vi "Local MS Auto.vi"() -> ()   [LabVIEW 2016]
uses:
  <vilib>/Platform/TimedLoop/XDataNode/timing_clust.ctl
  <vilib>/Platform/TimedLoop/XDataNode/nitl_modes.ctl
  <vilib>/Platform/TimedLoop/XDataNode/wakeup.ctl
  Subsystems/Global Variables.vi
  <vilib>/FPGAPlugInAG/PXI-7833R/niLvFpga_Open_PXI-7833R.vi
  <vilib>/Utility/error.llb/Error Cluster From Error Code.vi
  <vilib>/rvi/errors/niLvFpgaAdjustHostInterfaceError.vi
  <vilib>/FPGAPlugInAG/PXI-7833R/niLvFpga_Reset_PXI-7833R.vi
  <vilib>/FPGAPlugInAG/PXI-7833R/niLvFpga_Close_PXI-7833R.vi
  <vilib>/rvi/interface/nirviOpenFPGA/nirviOpenFPGA.xnode
  FPGA Bitfiles/PhantomControlPI_FPGATarget_QuadCtr2_E2412E44.lvbitx
  IRISS_FPGA_IO.vi
  <vilib>/rvi/interface/nirviReadWriteControl/nirviReadWriteControl.xnode
  <vilib>/platform/TimedLoop/XDataNode/XDataNode.xnode
  <vilib>/rvi/interface/nirviMethod/nirviMethod.xnode
  <vilib>/rvi/interface/nirviCloseFPGA/nirviCloseFPGA.xnode
  Library/KevinLibraryAll/labview2011/kevLib2011.lvlib
  NiFpgaLv.dll
  <vilib>/Platform/TimedLoop/XDataNode/XDNodeRunTimeDep.lvlib
panel:
  out "Pressure Reading":dbl[](array[numeric]) caption="IOP Output [mmHg]"
  in  "Pause":bool caption="To M/S"
  out "Trajectory Cluster":T1
  out "Update Mdl & Traj":bool=TRUE
  out "Stage PID Cluster":T2={"Stage Z PID"={"Kp"=0.0005, "Kd"=0.001, "Ki"=0.0}, "Stage Y PID"={"Kp"=0.0003, "Kd"=0.01, "Ki"=0.0}, "Stage X PID"={"Kp"=0.0003, "Kd"=0.01, "Ki"=0.0}}
  out "L1 to L4 PID Cluster":T3={"L1 PID Gains"={"Kp"=0.005, "Kd"=0.5, "Ki"=0.0005}, "L2 PID Gains"={"Kp"=0.01, "Kd"=1.0, "Ki"=0.0005}, "L3 PID Gains"={"Kp"=0.05, "Kd"=1.0, "Ki"=0.0005}, "L4 PID Gains"={"Kp"=0.1, "Kd"=1.0, "Ki"=0.0005}}
  in  "IRISS GUI":T4(tab)
  in  "OCT Direction":bool
  out "OCT Z out [mm]":dbl caption="OCT Out Z [mm]" format="%#.4f"
  out "X Stage out [mm] 2":dbl caption="Stage X [mm]" format="%#.4f"
  out "Z Stage out [mm] 2":dbl caption="Stage Z [mm]" format="%#.4f"
  out "Y Stage out [mm] 2":dbl caption="Stage Y [mm]" format="%#.4f"
  out "Vacuum Force [mmHg]  2":i32 caption="[mmHg]"
  out "Finished Late Counts":u16
  in  "L2 PID Gains":cluster{"Kp":dbl, "Kd":dbl, "Ki":dbl}={"Kp"=0.01, "Kd"=1.0, "Ki"=0.005}
  in  "L3 PID Gains":cluster{"Kp":dbl, "Kd":dbl, "Ki":dbl}={"Kp"=0.05, "Kd"=1.0, "Ki"=0.0005}
  in  "L4 PID Gains":cluster{"Kp":dbl, "Kd":dbl, "Ki":dbl}={"Kp"=0.1, "Kd"=0.1, "Ki"=0.0005}
  in  "L1 PID Gains":cluster{"Kp":dbl, "Kd":dbl, "Ki":dbl}={"Kp"=0.01, "Kd"=0.5, "Ki"=0.001}
  out "Current System State":T5(ring)
  out "State changing":bool
  out "Tip out Posit":dbl[](array[numeric]) caption="Position [mm]" format="%#.3f"
  out "Tip cmd Posit":dbl[](array[numeric]) caption="Command [mm]" format="%#.3f"
  out "L4 out Posit":dbl caption="y [deg]" format="%#.2g"
  out "L4 cmd Posit":dbl caption="r [deg]" format="%#.2g"
  out "L3 out Posit":dbl caption="y [mm]" format="%#.2g"
  out "L3 cmd Posit":dbl caption="r [mm]" format="%#.2g"
  out "L2 out Posit":dbl caption="y [deg]" format="%#.2g"
  out "L2 cmd Posit":dbl caption="r [deg]" format="%#.2g"
  out "L1 out Posit":dbl caption="y [deg]" format="%#.2g"
  out "L1 cmd Posit":dbl caption="r [deg]" format="%#.2g"
  out "State Flag Array":bool[](array[boolean])
  out "Irrigation Engaged? 2":bool caption="Irrigation Engaged"
  out "OCT Z cmd [mm]":dbl=6.0 caption="OCT Z Ref [mm]" min=0.0 max=12.0 step=0.5
  in  "OCT Z PID Gains":cluster{"Kp":dbl, "Kd":dbl, "Ki":dbl}={"Kp"=0.0003, "Kd"=0.0001, "Ki"=0.01}
  in  "L1 [deg]":dbl
  in  "L2 [deg]":dbl
  in  "L3 [mm]":dbl step=0.1
  in  "L4 [deg]":dbl
  in  "OCT Cmd  [mm]":dbl
  out "Current No.":u8
  in  "No. Cycles":u8=1
  in  "Joint Limits":dbl[][](array[numeric])=[[-8.0, 50.0], [-35.0, 35.0], [-5.0, 20.0], [-180.0, 180.0]] format="%#.3g"
  out "First Trk Pt":dbl[](array[numeric]) format="%#.3g"
  in  "Offset Home 2 RCM":dbl[](array[numeric])=[-7.7, 37.0, 55.0, 0.0] format="%#.3g"
  out "Error(s) Out on Program End":errorcluster
  out "L4 Chart":dbl(graph)
  out "L3 Chart":dbl(graph)
  out "L2 Chart":dbl(graph)
  out "L1 Chart":dbl(graph)
  out "Vac Input":sgl
  in  "Vacuum Step":bool
  in  "Clear Charts":bool
  out "AC Pressure [mmHg]":sgl
  in  "Take IOP Data":bool
  in  "Irrigation":bool
  in  "PID ON/OFF":bool
  in  "Vac PID Gains":cluster{"Kp":dbl, "Kd":dbl, "Ki":dbl, "Ts":dbl}={"Kp"=5.0, "Kd"=0.0, "Ki"=5.0, "Ts"=0.01}
  in  "Vac Cmd":sgl min=0 max=100 step=1 format="%#_13g"
  in  "Target IOP":sgl=20.0 min=0 max=100 step=1 format="%#_13g"
  out "IOP Ctrl":T6(graph)
  out "Pressure Sensors":T7(graph)
  in  "Reset Joystick":bool caption="Encoder Reset"
  in  "Max Limit [mmHg]":dbl=600.0
  in  "Increase":bool
  in  "Vac Step Size":sgl=50.0 min=0 max=100 step=1 format="%#_13g"
  in  "Wait Time [ms]":i32=200
  out "Vacuum":sgl
  out "Irrigation":sgl
  in  "Hydration":bool
  out "Z Stage out [mm]":dbl caption="Output Z [mm]" format="%#.4f"
  out "Z Stage cmd [mm]":dbl=6.0 caption="Reference Z [mm]" min=0.0 max=12.0 step=0.5
  out "Y Stage out [mm]":dbl caption="Output Y [mm]" format="%#.4f"
  out "Y Stage cmd [mm]":dbl=6.0 caption="Reference Y  [mm]" min=0.0 max=12.0 step=0.5
  out "X Stage out [mm]":dbl caption="Output X [mm]" format="%#.4f"
  out "X Stage cmd [mm]":dbl=6.0 caption="Reference X [mm]" min=0.0 max=12.0 step=0.5
  in  "Stage Z PID Gains":cluster{"Kp":dbl, "Kd":dbl, "Ki":dbl}={"Kp"=0.0005, "Kd"=0.001, "Ki"=0.0}
  in  "Stage Y PID Gains":cluster{"Kp":dbl, "Kd":dbl, "Ki":dbl}={"Kp"=0.0001, "Kd"=0.005, "Ki"=0.0}
  in  "Stage X PID Gains":cluster{"Kp":dbl, "Kd":dbl, "Ki":dbl}={"Kp"=0.0003, "Kd"=0.01, "Ki"=0.0}
  out "Irrigation Engaged?":bool
  out "Accurus Button":bool[](array[boolean]) caption="Remote Button Command"
  out "Voltage Output Ch. B":dbl(graph)
  out "Voltage Output Ch. A":dbl(graph)
  out "Accurus Engaged?":bool
  out "Vacuum Force [mmHg]":i32
  in  "Load Traj":bool caption="To M/S"
  in  "Retract":bool caption="To M/S"
  in  "Stop Accurus":bool caption="To M/S"
  in  "L3 Go Home":bool caption="To M/S"
  in  "Track":bool caption="To M/S"
  in  "Program Stop":bool
  # "Robot Status"
  # "OCT"
  # "Tool Tip Location"
  # "L1"
  # "X\nY\nZ"
  # "X\nY\nZ"
  # "+"
  # "_"
  # "L2"
  # "Reserved"
  # "System Progress"
  # "L3"
  # "Homing finished"
  # "Reserved"
  # "M/S initialization finished"
  # "Trajecoty loading finished"
  # "L4"
  # "Tracking initialization finished"
  # "In Tracking"
  # "Notes: \n2. check state transition\n4. preview trajectory?"
  # "Vacuum"
  # "Joint Motion"
  # "Calibration"
  # "Space Deform Parameters"
  # "L1"
  # "[deg]"
  # "L2"
  # "[deg]"
  # "L3"
  # "[mm]"
  # "L4"
  # "[deg]"
  # "First Track Point"
  # "AC & PC Gap"
  # "L1"
  # "[deg]"
  # "L2"
  # "[deg]"
  # "L3"
  # "[mm]"
  # "L4"
  # "[deg]"
  # "Error Message"
  # "Tracking Joint Limits"
  # "Incision"
  # "Min."
  # "Max."
  # "L1"
  # "L1"
  # "[deg]"
  # "L2"
  # "L2"
  # "[deg]"
  # "L3"
  # "L3"
  # "[mm]"
  # "L4"
  # "L4"
  # "[deg]"
  # "Data Saving"
  # "Vacuum Profile"
  # "IOP Feedback Control"
  # "Eye Hydration"
  # "XYZ Stage Control"
  # "OCT Z-Axis"
  # "Moved to main tab"
  # "Foot Pedal Buttons"
  # "Irrigation and Aspiration"
  # "Button 1"
  # "Button 2"
  # "Button 3"
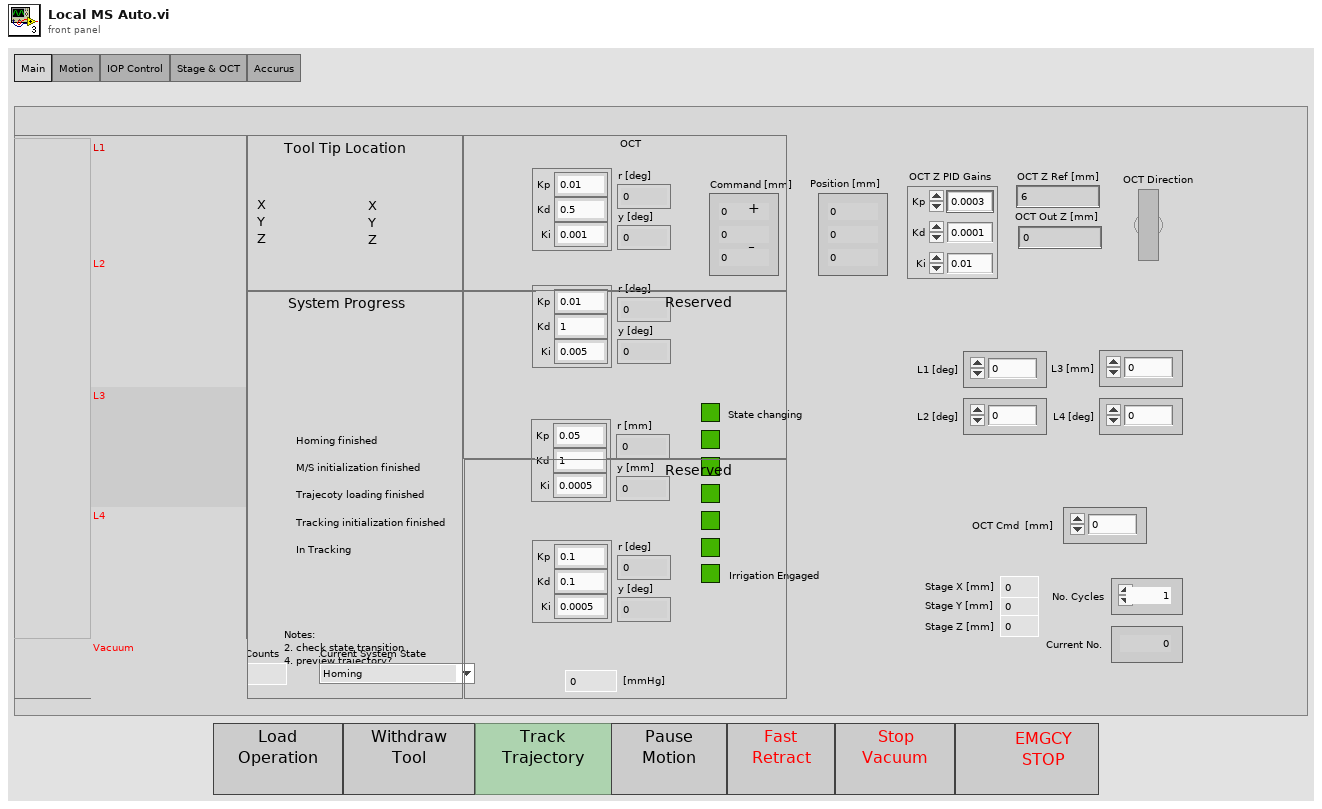
[diagram p1: front panel]
types:
  T1 = cluster{"Traj Px Array":dbl[], "Traj Py Array":dbl[], "Traj Pz Array":dbl[]}
  T2 = cluster{"Stage Z PID":cluster{"Kp":dbl, "Kd":dbl, "Ki":dbl}, "Stage Y PID":cluster{"Kp":dbl, "Kd":dbl, "Ki":dbl}, "Stage X PID":cluster{"Kp":dbl, "Kd":dbl, "Ki":dbl}}
  T3 = cluster{"L1 PID Gains":cluster{"Kp":dbl, "Kd":dbl, "Ki":dbl}, "L2 PID Gains":cluster{"Kp":dbl, "Kd":dbl, "Ki":dbl}, "L3 PID Gains":cluster{"Kp":dbl, "Kd":dbl, "Ki":dbl}, "L4 PID Gains":cluster{"Kp":dbl, "Kd":dbl, "Ki":dbl}}
  T4 = enum32{"Main", "Motion", "IOP Control", "Stage & OCT", "Accurus"}
  T5 = enum16{"Homing", "M/S Initialization", "M/S Operation", "Trajectory Loading", "Tracking Initialization", "Tracking"}
  T6 = cluster{"[0]":dbl, "[1]":dbl, "[2]":dbl, "[3]":dbl, "[4]":dbl, "[5]":dbl, "[6]":dbl, "[7]":dbl, "[8]":dbl}
  T7 = cluster{"Pressure Reading[0]":dbl, "Pressure Reading[1]":dbl, "Pressure Reading[2]":dbl, "Pressure Reading[3]":dbl, "Pressure Reading[4]":dbl, "Pressure Reading[5]":dbl, "Pressure Reading[6]":dbl, "Pressure Reading[7]":dbl, "Pressure Reading[8]":dbl}
  T8 = cluster{"Prev L1 to L4 Posit":dbl[], "Prev Stage Posit":dbl[], "Prev OCT Z Posit":dbl}
  T9 = typedef "XDNodeRunTimeDep.lvlib/timing_clust.ctl" = cluster{"Expected End [f-1]":u64, "Actual End [f-1]":u64, "Finished Late? [f-1]":bool, "Expected End [i-1]":u64, "Actual End [i-1]":u64, "Finished Late? [i-1]":bool, "Expected Start [i]":u64, "Actual Start [i]":u64, "Expected Start [f]":u64, "Actual Start [f]":u64, "Source Name":string, "Structure Name":string, "Period":i64, "Deadline":i64, "Offset":i64, "Start":i64, "Priority":i32, "Timeout":i32, "Mode":T10, "Wakeup Reason":T11, "Error":errorcluster, "Source Type":string, "Secondary Source Type":string, "Global End Time":u64, "Global Start Time":u64, "Frame Duration":u64, "Iteration Duration":u64, "Assigned CPU":i32, "I/O Scan Engine Mode":u32}
  T10 = typedef "XDNodeRunTimeDep.lvlib/nitl_modes.ctl" = enum32{"No Change", "Process missed periods, maintain original phase", "Discard missed periods, maintain original phase", "Process missed periods, ignore original phase", "Discard missed periods, ignore original phase"}
  T11 = typedef "XDNodeRunTimeDep.lvlib/wakeup.ctl" = enum32{"Normal", "Aborted", "Asynchronous wakeup", "Timing source error", "Timed loop error", "Timeout"}
  T12 = cluster{"L1 to L4 PID Cluster":cluster{"L1 PID Gains":cluster{"Kp":dbl, "Kd":dbl, "Ki":dbl}, "L2 PID Gains":cluster{"Kp":dbl, "Kd":dbl, "Ki":dbl}, "L3 PID Gains":cluster{"Kp":dbl, "Kd":dbl, "Ki":dbl}, "L4 PID Gains":cluster{"Kp":dbl, "Kd":dbl, "Ki":dbl}}, "Stage PID Cluster":cluster{"Stage Z PID":cluster{"Kp":dbl, "Kd":dbl, "Ki":dbl}, "Stage Y PID":cluster{"Kp":dbl, "Kd":dbl, "Ki":dbl}, "Stage X PID":cluster{"Kp":dbl, "Kd":dbl, "Ki":dbl}}, "OCT Z PID Gains":cluster{"Kp":dbl, "Kd":dbl, "Ki":dbl}}
  T13 = enum8{"Enabled", "Disabled", "Disabled and Grayed Out"}
  T14 = cluster{"Last L1 to L4 Posit":dbl[], "Last Stage Posit":dbl[], "Last OCT Z Posit":dbl}
  T15 = cluster{"Accurus button":bool[], "Accurus engaged?":bool, "Vacuum Force":i32, "Accurus Ch. A Vout":dbl, "Accurus Ch. B Vout":dbl, "Irrigation engaged?":bool}
  T16 = cluster{"pressure sensors[0]":sgl, "pressure sensors[1]":sgl, "pressure sensors[2]":sgl, "pressure sensors[3]":sgl, "pressure sensors[4]":sgl, "pressure sensors[5]":sgl, "pressure sensors[6]":sgl, "pressure sensors[7]":sgl, "pressure sensors[8]":sgl}[]
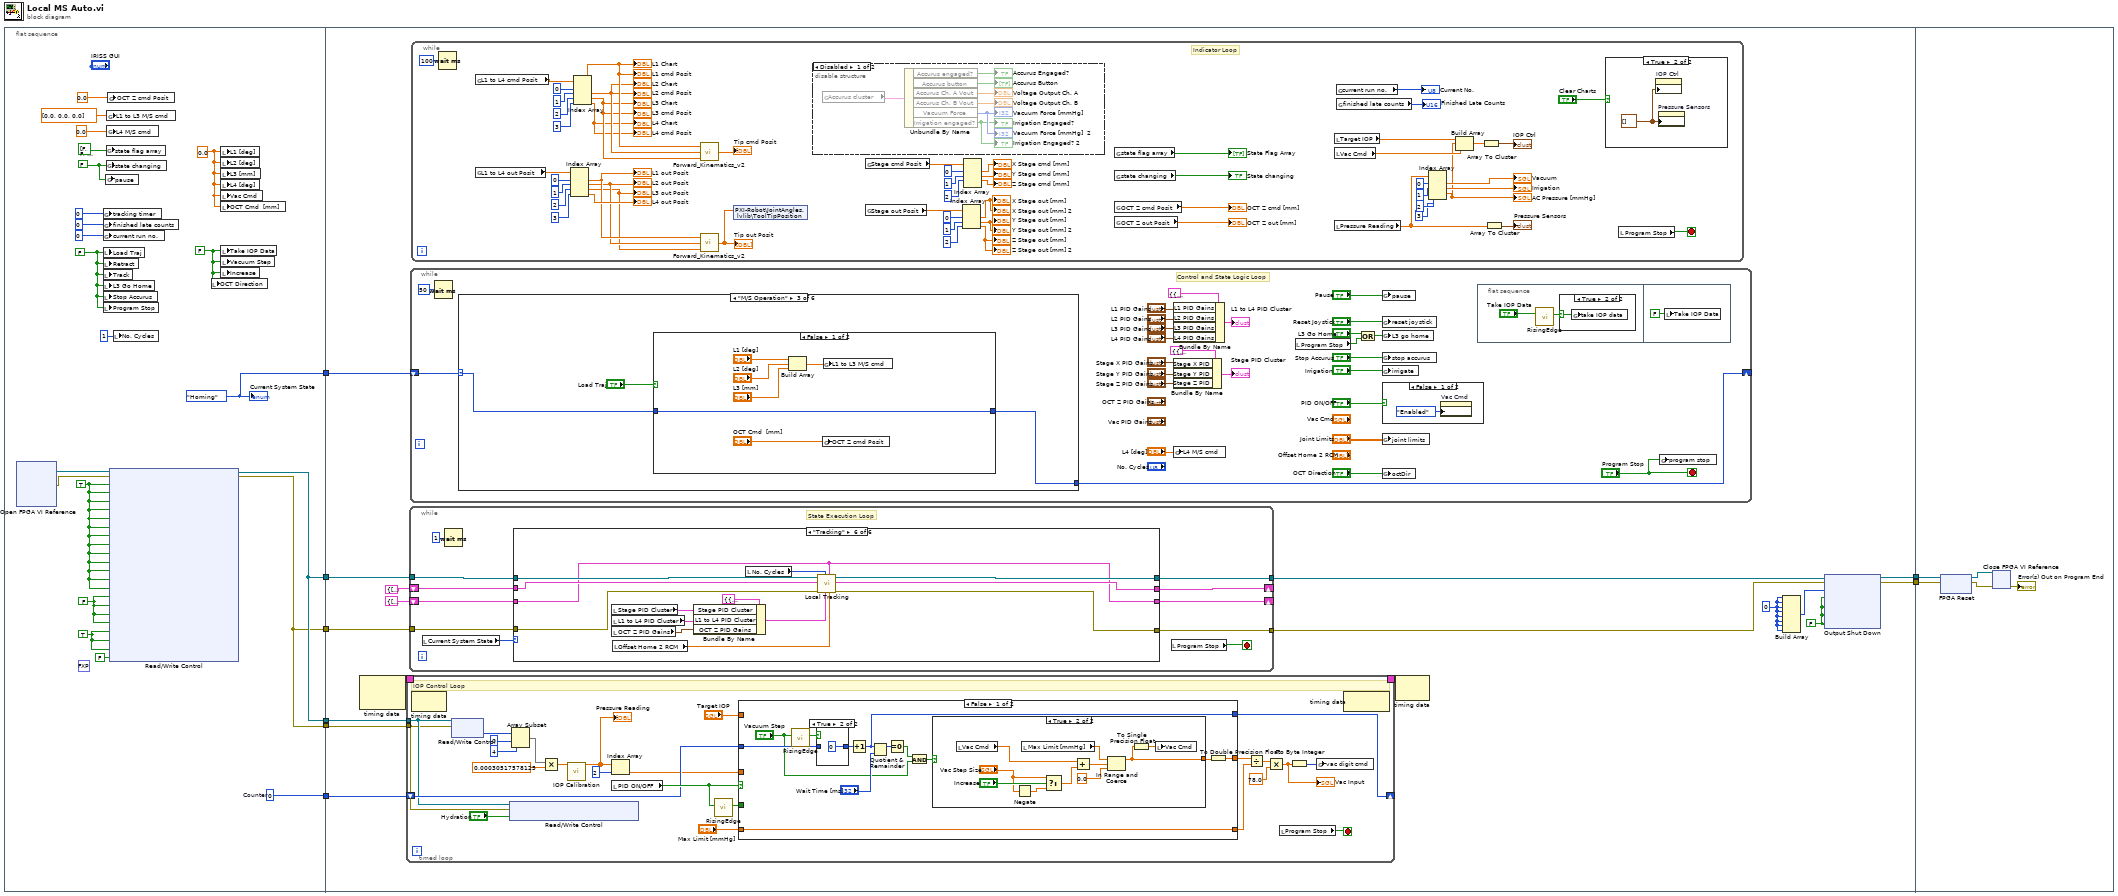
[diagram p0: block diagram]
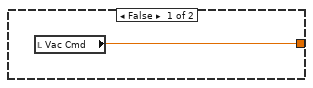
[diagram p3: hidden frame]
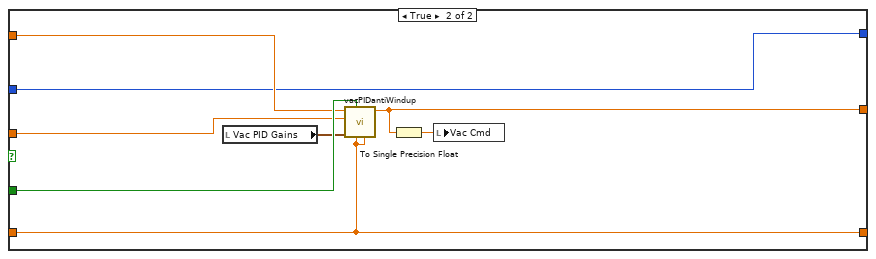
[diagram p4: hidden frame]
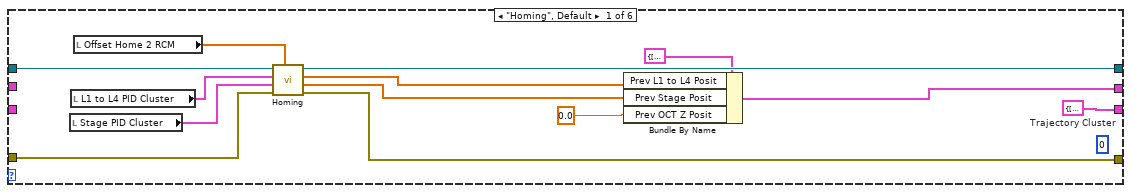
[diagram p7: hidden frame]
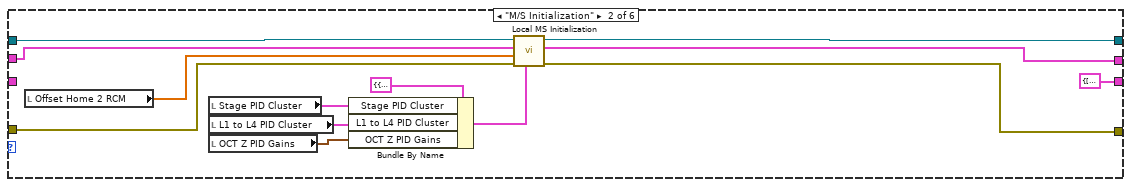
[diagram p8: hidden frame]
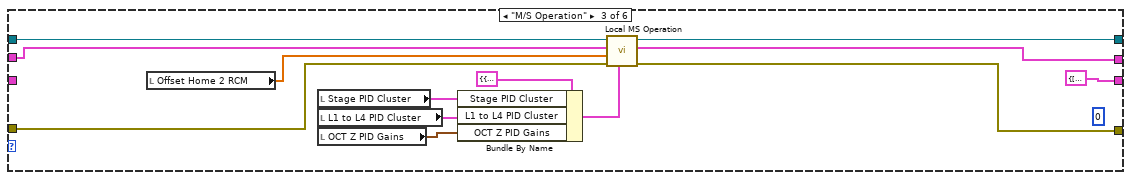
[diagram p9: hidden frame]
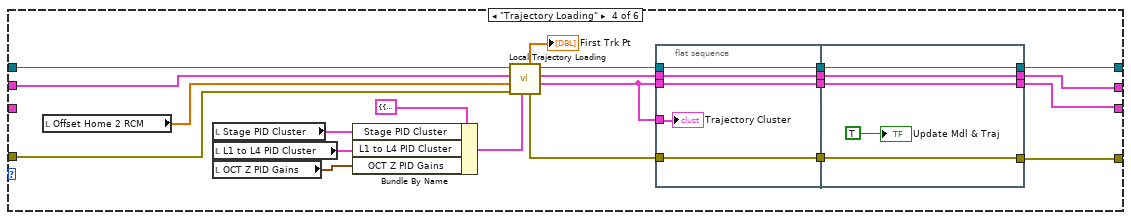
[diagram p10: hidden frame]
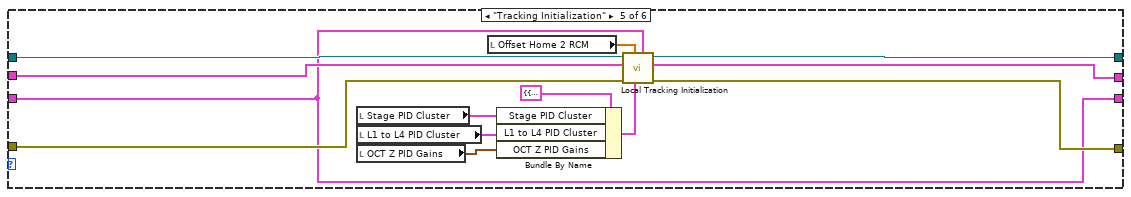
[diagram p11: hidden frame]
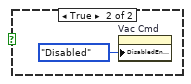
[diagram p13: hidden frame]
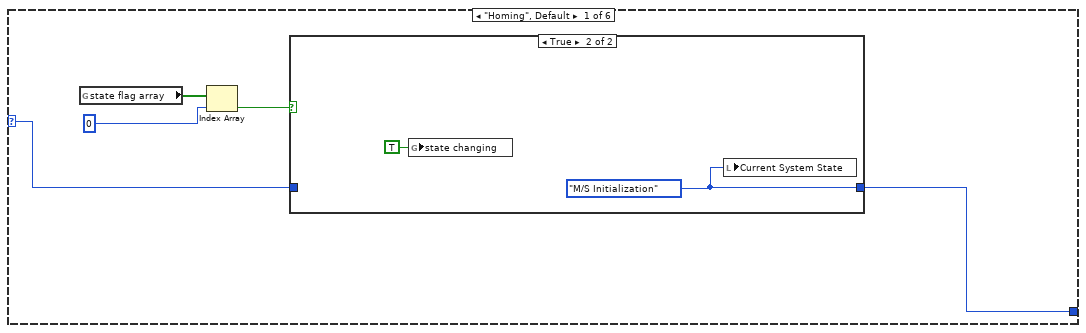
[diagram p14: hidden frame]
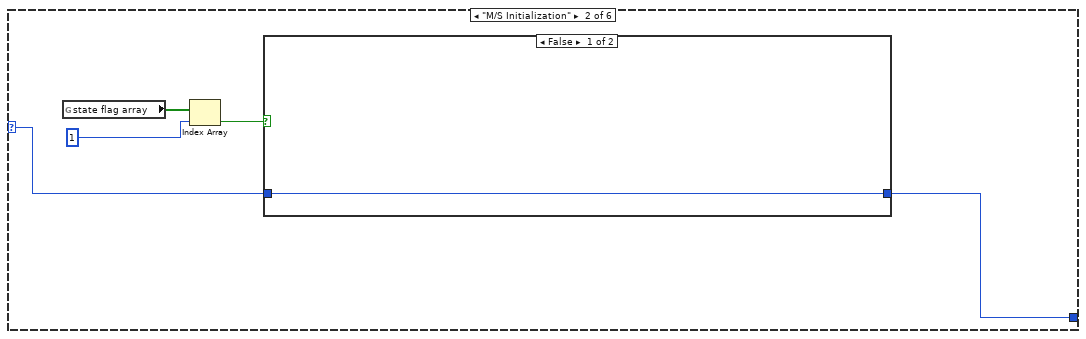
[diagram p16: hidden frame]
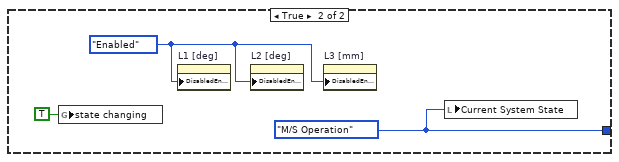
[diagram p17: hidden frame]
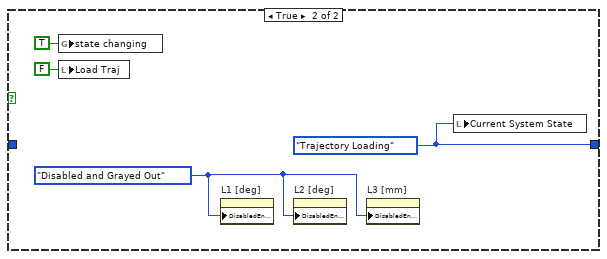
[diagram p18: hidden frame]
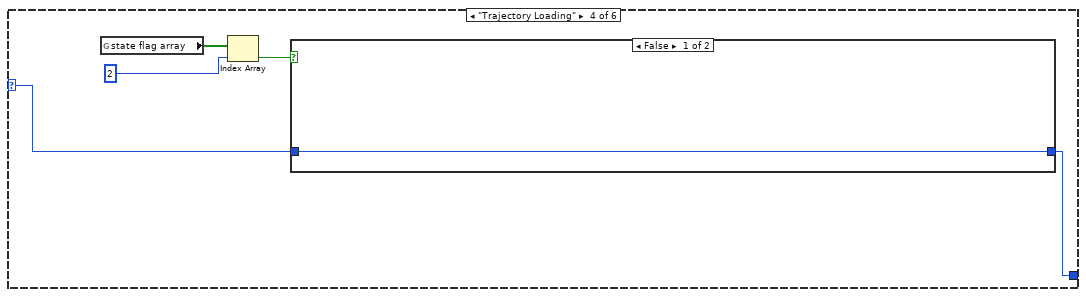
[diagram p19: hidden frame]
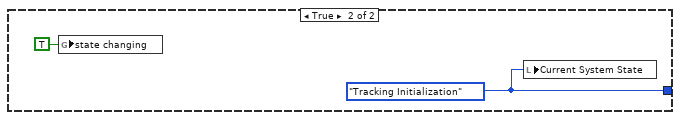
[diagram p20: hidden frame]
diagram:
  n1 = flat-sequence {
    tunnel: [w9] -> w8
    tunnel: [w10] -> w7
    tunnel: [w22] -> w6
    tunnel: [w10] -> w3
    tunnel: [w9] -> w2
    tunnel: [w14] -> w1
    tunnel: w8 -> [w46]
    tunnel: w7 -> [w47]
    tunnel: w6 -> [w38]
    tunnel: [w40] -> w5
    tunnel: [w39] -> w4
    tunnel: w3 -> [w33]
    tunnel: w2 -> [w32]
    tunnel: w1 -> [w31]
    tunnel: w5 -> [w395]
    tunnel: w4 -> [w396]
    frame #0 {
      (unwired) fxp<+,32,0> 0.0 ("Duty Cycle")
      w14 = 0  # Counter
      w11 = FALSE ("Take IOP Data")
      w12 = 0.0 ("L4 M/S cmd")
      w22 = T5."Homing" ("Current State")
      w23 = FALSE ("state changing")
      w29 = TRUE ("Conn0/DIO12 Button 1")
      w28 = FALSE ("Reset")
      w30 = TRUE ("Reset")
      w24 = FALSE ("program stop")
      n2 = xnode "Open FPGA VI Reference"() -> ("FPGA VI Reference Out"=w27:refnum<k20>, "error out"=w26:errorcluster)  [unwired: 2 in]
      n3 = global write "Global Variables.vi" "tracking timer"(0 ("finished late counts")) -> ()
      n4 = global write "Global Variables.vi" "finished late counts"(u16 0 ("finished late counts")) -> ()
      n5 = global write "Global Variables.vi" "current run no."(u8 0 ("current run no.")) -> ()
      n6 = local write "Load Traj"(w24) -> ()
      n7 = local write "Retract"(w24) -> ()
      n8 = local write "Track"(w24) -> ()
      n9 = local write "L3 Go Home"(w24) -> ()
      n10 = local write "Stop Accurus"(w24) -> ()
      n11 = local write "Program Stop"(w24) -> ()
      n12 = global write "Global Variables.vi" "pause"(w23) -> ()
      n13 = global write "Global Variables.vi" "state flag array"(bool[] [FALSE, FALSE, FALSE, FALSE, FALSE, FALSE, FALSE, FALSE, FALSE] ("state flag array")) -> ()
      n14 = global write "Global Variables.vi" "state changing"(w23) -> ()
      n15 = global write "Global Variables.vi" "L1 to L3 M/S cmd"(dbl[] [0.0, 0.0, 0.0] ("L1 to L3 M/S cmd")) -> ()
      n16 = global write "Global Variables.vi" "L4 M/S cmd"(0.0 ("L4 M/S cmd")) -> ()
      n17 = global write "Global Variables.vi" "OCT Z cmd Posit"(0.0 ("L4 M/S cmd")) -> ()
      n18 = xnode "Read/Write Control"("FPGA VI Reference In"=w27, "error in"=w26, "Reset 1"=w30, "Reset 3"=w30, "Reset 9"=w30, "Reset 10"=w30, "Reset 11"=w30, "Reset 12"=w30, "Reset 13"=w30, "Reset 14"=w30, "Reset 15"=w30, "Reset 16"=w30, "Reset 17"=w30, "Reset C1-1"=w30, "Reset C1-4"=w30, "INHB X"=w28, "INHB Y"=w28, "INHB Z"=w28, "INHB OCT Mot"=w28, "Conn0/DIO12 Button 1"=w29, "Conn0/DIO13 Button 2"=w29, "Conn0/DIO15 Button 4"=w29, "Hydration On/Off (Connector2/DIO28)"=FALSE) -> ("FPGA VI Reference Out"=w10:refnum<k20>, "error out"=w9:errorcluster)
      n19 = local write "No. Cycles"(1 ("No. Cycles")) -> ()
      n20 = local write "OCT Direction"(w11) -> ()
      n21 = local write "L1 [deg]"(w12) -> ()
      n22 = local write "L2 [deg]"(w12) -> ()
      n23 = local write "L3 [mm]"(w12) -> ()
      n24 = local write "L4 [deg]"(w12) -> ()
      n25 = local write "Vac Cmd"(w12) -> ()
      n26 = local write "OCT Cmd  [mm]"(w12) -> ()
      n27 = local write "Take IOP Data"(w11) -> ()
      n28 = local write "Vacuum Step"(w11) -> ()
      n29 = local write "Increase"(w11) -> ()
      "Current System State" <- w22
    }
    frame #1 {
      w44 = FALSE
      w37 = i16 0 ("element")
      n30 = node-c288 ("Input Node")() -> (w35:T9)  [unwired: 2 in]
      n31 = timed-loop {
        timing: w35 -> [_]
        timing-out: [_] -> w34
        tunnel: w33 -> [w50]
        tunnel: w32 -> [w49]
        shift-right: [w52] -> _
        shift-left: w31 -> [w53]
        stop <- w63 stop-if-true
        # "IOP Control Loop"
        n32 = node-c288() -> ()  [unwired: 1 in, 1 out]
        n33 = xnode "Read/Write Control"("FPGA VI Reference In"=w50, "error in"=w49) -> ("AI"=w66:i16[])  [unwired: 2 out]
        n34 = xnode "Read/Write Control"("FPGA VI Reference In"=w50, "error in"=w49, "Hydration On/Off (Connector2/DIO28)"="Hydration") -> ()  [unwired: 2 out]
        n35 = Array Subset(array=w66, index=0, length=4) -> (w72:i16[])
        n36 = Multiply(x=w72, y=0.00030517578125) -> (x*y=w56:dbl[])
        n37 = call "IOP Calibration.vi"("IOP Input [V]"=w56) -> ("IOP Output [mmHg]"=w67:dbl[])  [unwired: 10 in]
        "Pressure Reading" <- w67
        n38 = Index Array(array=w67, index=2) -> (element=w48:dbl)
        n39 = local read "PID ON/OFF"() -> (w64:bool)
        n40 = call "RisingEdge.vi"("Signal In"=w64) -> ("Rising Edge"=w65:bool)  [unwired: 10 in]
        n41 = case shown="False" w64 {
          tunnel: w48 -> [_ w101]
          tunnel: "Target IOP" -> [_ w102]
          tunnel: [w84 w105] -> w62
          tunnel: "Max Limit [mmHg]" -> [w83 w104]
          tunnel: [w83 w104] -> w54
          tunnel: w65 -> [_ w103]
          tunnel: w53 -> [w76 w98]
          tunnel: [w73 w98] -> w52
          frame False {
            n42 = call "RisingEdge.vi"("Signal In"="Vacuum Step") -> ("Rising Edge"=w77:bool)  [unwired: 10 in]
            n43 = case shown="True" w77 {
              tunnel: [w85 0] -> w80
              tunnel: w76 -> [w85 _]
              frame False {
              }
              frame True {
              }
            }
            n44 = Increment(x=w80) -> (x+1=w73:i32)
            n45 = Quotient & Remainder(x=w73, y="Wait Time [ms]") -> (x-y*floor(x/y)=w79:i32)  [unwired: 1 out]
            n46 = Equal To 0?(x=w79) -> (x = 0?=w81:bool)
            n47 = And(x=w81, y="Vacuum Step") -> (x .and. y?=w75:bool)
            n48 = case shown="True" w75 {
              tunnel: [w87 w97] -> w82
              frame False {
                n49 = local read "Vac Cmd"() -> (w87:sgl)
              }
              frame True {
                n50 = local read "Vac Cmd"() -> (w90:sgl)
                n51 = Negate(x="Vac Step Size") -> (-x=w88:sgl)
                n52 = local read "Max Limit [mmHg]"() -> (w94:dbl)
                n53 = Select(t="Vac Step Size", s="Increase", f=w88) -> (s? t:f=w92:sgl)
                n54 = Add(x=w90, y=w92) -> (x+y=w96:sgl)
                n55 = In Range and Coerce(upper limit=w94, x=w96, lower limit=0.0 ("y")) -> (coerced(x)=w97:dbl)  [unwired: 1 out]
                n56 = To Single Precision Float(number=w97) -> (single precision float=w91:sgl)
                n57 = local write "Vac Cmd"(w91) -> ()
              }
            }
            n58 = To Double Precision Float(number=w82) -> (double precision float=w84:dbl)
          }
          frame True {
            n59 = local read "Vac PID Gains"() -> (w100:cluster{"Kp":dbl, "Kd":dbl, "Ki":dbl, "Ts":dbl})
            n60 = call "vacPIDantiWindup.vi"("Saturation U"=w104, "Saturation M"=w104, "Reset"=w103, "PID Gains"=w100, "Feedback"=w101, "Reference"=w102) -> ("Control"=w105:dbl)  [unwired: 5 in]
            n61 = To Single Precision Float(number=w105) -> (single precision float=w99:sgl)
            n62 = local write "Vac Cmd"(w99) -> ()
          }
        }
        n63 = Divide(x=w62, y=w54) -> (x/y=w61:dbl)
        n64 = Multiply(x=w61, y=78.0) -> (x*y=w55:dbl)
        "Vac Input" <- w55
        n65 = local read "Program Stop"() -> (w63:bool)
        n66 = To Byte Integer(number=w55) -> (8bit integer=w59:i8)
        n67 = global write "Global Variables.vi" "vac digit cmd"(w59) -> ()
        n68 = node-c288() -> ()  [unwired: 1 in, 1 out]
      }
      n69 = while {
        tunnel: w47 -> [w182]
        tunnel: w46 -> [w181]
        tunnel: [w180] -> w42
        tunnel: [w179] -> w41
        shift-right: [w177] -> _
        shift-left: T8 {"Prev L1 to L4 Posit"=[0.0, 0.0, 0.0, 0.0], "Prev Stage Posit"=[6.0, 6.0, 6.0], "Prev OCT Z Posit"=0.0} ("Prev Posit Cluster") -> [w178]
        shift-right: [w175] -> _
        shift-left: T1 {"Traj Px Array"=[], "Traj Py Array"=[], "Traj Pz Array"=[]} ("Trajectory Cluster") -> [w174]
        stop <- w176 stop-if-true
        # "State Execution Loop"
        n70 = local read "Current System State"() -> (w183:T5)
        n71 = Wait (ms)(milliseconds to wait=u32 1) -> ()  [unwired: 1 out]
        n72 = case shown="\"Tracking\"" w183 {
          tunnel: w182 -> [w197 w210 w223 w245 w268 w282]
          tunnel: w181 -> [w196 w209 w222 w244 w267 w281]
          tunnel: [w195 w208 w221 w227 w266 w280] -> w180
          tunnel: [w194 w207 w220 w233 w265 w279] -> w179
          tunnel: w178 -> [_ w206 w219 w243 w263 w278]
          tunnel: [w193 w205 w218 w232 w264 w277] -> w177
          tunnel: [w185 T1 {"Traj Px Array"=[], "Traj Py Array"=[], "Traj Pz Array"=[]} ("Trajectory Cluster") T1 {"Traj Px Array"=[], "Traj Py Array"=[], "Traj Pz Array"=[]} ("Trajectory Cluster") w225 w256 w271] -> w175
          tunnel: w174 -> [_ _ _ _ w256 w271]
          frame "Homing", Default {
            w185 = T1 {"Traj Px Array"=[], "Traj Py Array"=[], "Traj Pz Array"=[]}  # Trajectory Cluster
            (unwired) 0 ("Last Index")
            n73 = local read "Stage PID Cluster"() -> (w189:T2)
            n74 = local read "L1 to L4 PID Cluster"() -> (w190:T3)
            n75 = local read "Offset Home 2 RCM"() -> (w192:dbl[])
            n76 = call "Homing.vi"("Offset Home 2 RCM"=w192, "error in"=w196, "Stage PID Cluster"=w189, "L1 to L4 PID Cluster"=w190, "FPGA VI Reference In"=w197) -> ("error out"=w194:errorcluster, "Last Stage Posit"=w186:dbl[], "Last L1 to L4 Posit"=w187:dbl[], "FPGA VI Reference Out"=w195:refnum<k20>)  [unwired: 3 in]
            n77 = Bundle By Name(cluster=T8 {"Prev L1 to L4 Posit"=[-0.5409, 0.04404050915429177, -1.917656453185038, 0.02068014705882353], "Prev Stage Posit"=[6.001471972029684, 5.996134588585126, 6.000298217087839], "Prev OCT Z Posit"=-0.0} ("Prev Posit Cluster"), "Prev L1 to L4 Posit"=w187, "Prev Stage Posit"=w186, "Prev OCT Z Posit"=0.0) -> (w193:T8)
          }
          frame "M/S Initialization" {
            n78 = local read "Offset Home 2 RCM"() -> (w199:dbl[])
            n79 = local read "Stage PID Cluster"() -> (w204:T2)
            n80 = local read "L1 to L4 PID Cluster"() -> (w203:T3)
            n81 = local read "OCT Z PID Gains"() -> (w202:cluster{"Kp":dbl, "Kd":dbl, "Ki":dbl})
            n82 = Bundle By Name(cluster=T12 {"L1 to L4 PID Cluster"={"L1 PID Gains"={"Kp"=0.005, "Kd"=0.5, "Ki"=0.0005}, "L2 PID Gains"={"Kp"=0.01, "Kd"=1.0, "Ki"=0.005}, "L3 PID Gains"={"Kp"=0.05, "Kd"=1.0, "Ki"=0.0005}, "L4 PID Gains"={"Kp"=0.1, "Kd"=0.1, "Ki"=0.0005}}, "Stage PID Cluster"={"Stage Z PID"={"Kp"=0.0005, "Kd"=0.001, "Ki"=0.0}, "Stage Y PID"={"Kp"=0.0003, "Kd"=0.01, "Ki"=0.0}, "Stage X PID"={"Kp"=0.0003, "Kd"=0.01, "Ki"=0.0}}, "OCT Z PID Gains"={"Kp"=0.0003, "Kd"=0.0001, "Ki"=0.01}} ("PID Cluster"), "Stage PID Cluster"=w204, "L1 to L4 PID Cluster"=w203, "OCT Z PID Gains"=w202) -> (w200:T12)
            n83 = call "Local MS Initialization.vi"("PID Cluster"=w200, "error in"=w209, "Offset Home 2 RCM"=w199, "Prev Posit Cluster"=w206, "FPGA VI Reference In"=w210) -> ("error out"=w207:errorcluster, "Last Posit Cluster"=w205:T14, "FPGA VI Reference Out"=w208:refnum<k20>)  [unwired: 4 in]
          }
          frame "M/S Operation" {
            (unwired) 0 ("Last Index")
            n84 = local read "Offset Home 2 RCM"() -> (w212:dbl[])
            n85 = local read "Stage PID Cluster"() -> (w217:T2)
            n86 = local read "L1 to L4 PID Cluster"() -> (w216:T3)
            n87 = local read "OCT Z PID Gains"() -> (w215:cluster{"Kp":dbl, "Kd":dbl, "Ki":dbl})
            n88 = Bundle By Name(cluster=T12 {"L1 to L4 PID Cluster"={"L1 PID Gains"={"Kp"=0.005, "Kd"=0.5, "Ki"=0.0005}, "L2 PID Gains"={"Kp"=0.01, "Kd"=1.0, "Ki"=0.005}, "L3 PID Gains"={"Kp"=0.05, "Kd"=1.0, "Ki"=0.0005}, "L4 PID Gains"={"Kp"=0.1, "Kd"=0.1, "Ki"=0.0005}}, "Stage PID Cluster"={"Stage Z PID"={"Kp"=0.0005, "Kd"=0.001, "Ki"=0.0}, "Stage Y PID"={"Kp"=0.0003, "Kd"=0.01, "Ki"=0.0}, "Stage X PID"={"Kp"=0.0003, "Kd"=0.01, "Ki"=0.0}}, "OCT Z PID Gains"={"Kp"=0.0003, "Kd"=0.0001, "Ki"=0.01}} ("PID Cluster"), "Stage PID Cluster"=w217, "L1 to L4 PID Cluster"=w216, "OCT Z PID Gains"=w215) -> (w213:T12)
            n89 = call "Local MS Operation.vi"("PID Cluster"=w213, "error in"=w222, "Offset Home 2 RCM"=w212, "Prev Posit Cluster"=w219, "FPGA VI Reference In"=w223) -> ("error out"=w220:errorcluster, "Last Posit Cluster"=w218:T14, "FPGA VI Reference Out"=w221:refnum<k20>)  [unwired: 4 in]
          }
          frame "Trajectory Loading" {
            n90 = local read "Offset Home 2 RCM"() -> (w237:dbl[])
            n91 = local read "Stage PID Cluster"() -> (w242:T2)
            n92 = local read "L1 to L4 PID Cluster"() -> (w241:T3)
            n93 = local read "OCT Z PID Gains"() -> (w240:cluster{"Kp":dbl, "Kd":dbl, "Ki":dbl})
            n94 = Bundle By Name(cluster=T12 {"L1 to L4 PID Cluster"={"L1 PID Gains"={"Kp"=0.005, "Kd"=0.5, "Ki"=0.0005}, "L2 PID Gains"={"Kp"=0.01, "Kd"=1.0, "Ki"=0.005}, "L3 PID Gains"={"Kp"=0.05, "Kd"=1.0, "Ki"=0.0005}, "L4 PID Gains"={"Kp"=0.1, "Kd"=0.1, "Ki"=0.0005}}, "Stage PID Cluster"={"Stage Z PID"={"Kp"=0.0005, "Kd"=0.001, "Ki"=0.0}, "Stage Y PID"={"Kp"=0.0003, "Kd"=0.01, "Ki"=0.0}, "Stage X PID"={"Kp"=0.0003, "Kd"=0.01, "Ki"=0.0}}, "OCT Z PID Gains"={"Kp"=0.0003, "Kd"=0.0001, "Ki"=0.01}} ("PID Cluster"), "Stage PID Cluster"=w242, "L1 to L4 PID Cluster"=w241, "OCT Z PID Gains"=w240) -> (w238:T12)
            n95 = call "Local Trajectory Loading.vi"("PID Cluster"=w238, "error in"=w244, "Offset Home 2 RCM"=w237, "Prev Posit Cluster"=w243, "FPGA VI Reference In"=w245) -> ("Trajectory Cluster"=w224:T1, "Last Posit Cluster"=w231:T14, "FPGA VI Reference Out"=w229:refnum<k20>, "error out"=w235:errorcluster, "First Trk Pt"=→"First Trk Pt":dbl[])  [unwired: 2 in]
            n96 = flat-sequence {
              tunnel: w224 -> [w250]
              tunnel: w235 -> [w249]
              tunnel: [w249] -> w234
              tunnel: w231 -> [w248]
              tunnel: [w248] -> w230
              tunnel: w229 -> [w247]
              tunnel: [w247] -> w228
              tunnel: [w246] -> w226
              tunnel: w224 -> [w246]
              tunnel: [w254] -> w233
              tunnel: w234 -> [w254]
              tunnel: [w253] -> w232
              tunnel: w230 -> [w253]
              tunnel: w228 -> [w252]
              tunnel: [w252] -> w227
              tunnel: w226 -> [w251]
              tunnel: [w251] -> w225
              frame #0 {
                "Trajectory Cluster" <- w250
              }
              frame #1 {
                "Update Mdl & Traj" <- TRUE
              }
            }
          }
          frame "Tracking Initialization" {
            n97 = local read "Stage PID Cluster"() -> (w261:T2)
            n98 = local read "L1 to L4 PID Cluster"() -> (w260:T3)
            n99 = local read "OCT Z PID Gains"() -> (w258:cluster{"Kp":dbl, "Kd":dbl, "Ki":dbl})
            n100 = local read "Offset Home 2 RCM"() -> (w262:dbl[])
            n101 = Bundle By Name(cluster=T12 {"L1 to L4 PID Cluster"={"L1 PID Gains"={"Kp"=0.005, "Kd"=0.5, "Ki"=0.0005}, "L2 PID Gains"={"Kp"=0.01, "Kd"=1.0, "Ki"=0.005}, "L3 PID Gains"={"Kp"=0.05, "Kd"=1.0, "Ki"=0.0005}, "L4 PID Gains"={"Kp"=0.1, "Kd"=0.1, "Ki"=0.0005}}, "Stage PID Cluster"={"Stage Z PID"={"Kp"=0.0005, "Kd"=0.001, "Ki"=0.0}, "Stage Y PID"={"Kp"=0.0003, "Kd"=0.01, "Ki"=0.0}, "Stage X PID"={"Kp"=0.0003, "Kd"=0.01, "Ki"=0.0}}, "OCT Z PID Gains"={"Kp"=0.0003, "Kd"=0.0001, "Ki"=0.01}} ("PID Cluster"), "Stage PID Cluster"=w261, "L1 to L4 PID Cluster"=w260, "OCT Z PID Gains"=w258) -> (w257:T12)
            n102 = call "Local Tracking Initialization.vi"("Trajectory Cluster"=w256, "PID Cluster"=w257, "Offset Home 2 RCM"=w262, "error in"=w267, "Prev Posit Cluster"=w263, "FPGA VI Reference In"=w268) -> ("error out"=w265:errorcluster, "Last Posit Cluster"=w264:T14, "FPGA VI Reference Out"=w266:refnum<k20>)  [unwired: 3 in]
          }
          frame "Tracking" {
            n103 = local read "Stage PID Cluster"() -> (w276:T2)
            n104 = local read "L1 to L4 PID Cluster"() -> (w275:T3)
            n105 = local read "OCT Z PID Gains"() -> (w274:cluster{"Kp":dbl, "Kd":dbl, "Ki":dbl})
            n106 = local read "Offset Home 2 RCM"() -> (w270:dbl[])
            n107 = Bundle By Name(cluster=T12 {"L1 to L4 PID Cluster"={"L1 PID Gains"={"Kp"=0.005, "Kd"=0.5, "Ki"=0.0005}, "L2 PID Gains"={"Kp"=0.01, "Kd"=1.0, "Ki"=0.005}, "L3 PID Gains"={"Kp"=0.05, "Kd"=1.0, "Ki"=0.0005}, "L4 PID Gains"={"Kp"=0.1, "Kd"=0.1, "Ki"=0.0005}}, "Stage PID Cluster"={"Stage Z PID"={"Kp"=0.0005, "Kd"=0.001, "Ki"=0.0}, "Stage Y PID"={"Kp"=0.0003, "Kd"=0.01, "Ki"=0.0}, "Stage X PID"={"Kp"=0.0003, "Kd"=0.01, "Ki"=0.0}}, "OCT Z PID Gains"={"Kp"=0.0003, "Kd"=0.0001, "Ki"=0.01}} ("PID Cluster"), "Stage PID Cluster"=w276, "L1 to L4 PID Cluster"=w275, "OCT Z PID Gains"=w274) -> (w272:T12)
            n108 = local read "No. Cycles"() -> (w269:u8)
            n109 = call "Local Tracking.vi"("Offset Home 2 RCM"=w270, "Trajectory Cluster"=w271, "PID Cluster"=w272, "No. Cycles"=w269, "error in"=w281, "Prev Posit Cluster"=w278, "FPGA VI Reference In"=w282) -> ("error out"=w279:errorcluster, "Last Posit Cluster"=w277:T14, "FPGA VI Reference Out"=w280:refnum<k20>)  [unwired: 2 in]
          }
        }
        n110 = local read "Program Stop"() -> (w176:bool)
      }
      n111 = while {
        shift-right: [w289] -> _
        shift-left: w38 -> [w290]
        stop <- "Program Stop" stop-if-true
        # "Control and State Logic Loop"
        n112 = Wait (ms)(milliseconds to wait=u32 50) -> ()  [unwired: 1 out]
        n113 = case shown="\"M/S Operation\"" w290 {
          selector: w290 -> [w317 w323 w334 w345 w353 w382]
          tunnel: [w316 w324 w333 w346 w354 w383] -> w289
          frame "Homing", Default {
            n114 = global read "Global Variables.vi" "state flag array"() -> (w318:bool[])
            n115 = Index Array(array=w318, index=0) -> (element=w315:bool)
            n116 = case shown="True" w315 {
              tunnel: [w320 w321] -> w316
              tunnel: w317 -> [w320 _]
              frame False {
                # "homing in process"
              }
              frame True {
                w321 = T5."M/S Initialization" ("Current State")
                # "finish homing"
                n117 = global write "Global Variables.vi" "state changing"(TRUE ("state changing")) -> ()
                n118 = local write "Current System State"(w321) -> ()
              }
            }
          }
          frame "M/S Initialization" {
            n119 = global read "Global Variables.vi" "state flag array"() -> (w326:bool[])
            n120 = Index Array(array=w326, index=1) -> (element=w325:bool)
            n121 = case shown="False" w325 {
              tunnel: [w328 w330] -> w324
              tunnel: w323 -> [w328 _]
              frame False {
              }
              frame True {
                w330 = T5."M/S Operation" ("Current State")
                w329 = T13."Enabled" ("Disabled")
                n122 = global write "Global Variables.vi" "state changing"(TRUE ("state changing")) -> ()
                n123 = property on="L1 [deg]" class="DigNum (strict)"("DisabledEnum"=w329) -> ()  [unwired: 2 in, 2 out]
                n124 = property on="L2 [deg]" class="DigNum (strict)"("DisabledEnum"=w329) -> ()  [unwired: 2 in, 2 out]
                n125 = property on="L3 [mm]" class="DigNum (strict)"("DisabledEnum"=w329) -> ()  [unwired: 2 in, 2 out]
                n126 = local write "Current System State"(w330) -> ()
              }
            }
          }
          frame "M/S Operation" {
            n127 = case shown="False" "Load Traj" {
              tunnel: w334 -> [w340 _]
              tunnel: [w340 w342] -> w333
              frame False {
                n128 = Build Array("L1 [deg]", "L2 [deg]", "L3 [mm]") -> (w338:dbl[])
                n129 = global write "Global Variables.vi" "OCT Z cmd Posit"("OCT Cmd  [mm]") -> ()
                n130 = global write "Global Variables.vi" "L1 to L3 M/S cmd"(w338) -> ()
              }
              frame True {
                w342 = T5."Trajectory Loading" ("Current State")
                w341 = T13."Disabled and Grayed Out" ("Disabled")
                n131 = global write "Global Variables.vi" "state changing"(TRUE ("state changing")) -> ()
                n132 = local write "Load Traj"(FALSE ("Load Traj")) -> ()
                n133 = property on="L1 [deg]" class="DigNum (strict)"("DisabledEnum"=w341) -> ()  [unwired: 2 in, 2 out]
                n134 = property on="L2 [deg]" class="DigNum (strict)"("DisabledEnum"=w341) -> ()  [unwired: 2 in, 2 out]
                n135 = property on="L3 [mm]" class="DigNum (strict)"("DisabledEnum"=w341) -> ()  [unwired: 2 in, 2 out]
                n136 = local write "Current System State"(w342) -> ()
              }
            }
          }
          frame "Trajectory Loading" {
            n137 = global read "Global Variables.vi" "state flag array"() -> (w348:bool[])
            n138 = Index Array(array=w348, index=2) -> (element=w347:bool)
            n139 = case shown="False" w347 {
              tunnel: [w350 w351] -> w346
              tunnel: w345 -> [w350 _]
              frame False {
              }
              frame True {
                w351 = T5."Tracking Initialization" ("Current State")
                n140 = global write "Global Variables.vi" "state changing"(TRUE ("state changing")) -> ()
                n141 = local write "Current System State"(w351) -> ()
              }
            }
          }
          frame "Tracking Initialization" {
            n142 = global read "Global Variables.vi" "state flag array"() -> (w356:bool[])
            n143 = Index Array(array=w356, index=3) -> (element=w355:bool)
            n144 = case shown="True" w355 {
              tunnel: [w358 w368] -> w354
              tunnel: w353 -> [w359 w367]
              frame False {
                n145 = local read "Retract"() -> (w360:bool)
                n146 = case shown="False" w360 {
                  tunnel: w359 -> [w361 _]
                  tunnel: [w361 w364] -> w358
                  frame False {
                  }
                  frame True {
                    w364 = T5."M/S Initialization" ("Current State")
                    n147 = global write "Global Variables.vi" "state changing"(TRUE ("state changing")) -> ()
                    n148 = local write "Retract"(FALSE ("Load Traj")) -> ()
                    n149 = local write "Current System State"(w364) -> ()
                  }
                }
              }
              frame True {
                n150 = local read "Load Traj"() -> (w369:bool)
                n151 = Build Array("Track", w369, "Retract") -> (w371:bool[])
                n152 = Boolean Array To Number(Boolean array=w371) -> (number=w370:u32)
                n153 = case shown="2" w370 {
                  tunnel: [w372 w373 w376 w379] -> w368
                  tunnel: w367 -> [w372 _ _ _]
                  frame 0, Default {
                  }
                  frame 1 {
                    w373 = T5."Tracking" ("Current State")
                    n154 = global write "Global Variables.vi" "state changing"(TRUE ("state changing")) -> ()
                    n155 = local write "Track"(FALSE ("Track")) -> ()
                    n156 = local write "Current System State"(w373) -> ()
                  }
                  frame 2 {
                    w376 = T5."Trajectory Loading" ("Current State")
                    n157 = global write "Global Variables.vi" "state changing"(TRUE ("state changing")) -> ()
                    n158 = local write "Load Traj"(FALSE ("Load Traj")) -> ()
                    n159 = local write "Current System State"(w376) -> ()
                  }
                  frame 4 {
                    w379 = T5."M/S Initialization" ("Current State")
                    n160 = global write "Global Variables.vi" "state changing"(TRUE ("state changing")) -> ()
                    n161 = local write "Retract"(FALSE ("Load Traj")) -> ()
                    n162 = local write "Current System State"(w379) -> ()
                  }
                }
              }
            }
          }
          frame "Tracking" {
            n163 = global read "Global Variables.vi" "state flag array"() -> (w385:bool[])
            n164 = Index Array(array=w385, index=4) -> (element=w384:bool)
            n165 = case shown="True" w384 {
              tunnel: [w387 w390] -> w383
              tunnel: w382 -> [w387 w389]
              frame False {
              }
              frame True {
                n166 = local read "Retract"() -> (w388:bool)
                n167 = case shown="True" w388 {
                  tunnel: [w391 w392] -> w390
                  tunnel: w389 -> [w391 _]
                  frame False {
                  }
                  frame True {
                    w392 = T5."M/S Initialization" ("Current State")
                    n168 = global write "Global Variables.vi" "state changing"(TRUE ("state changing")) -> ()
                    n169 = local write "Retract"(FALSE ("Load Traj")) -> ()
                    n170 = local write "Current System State"(w392) -> ()
                  }
                }
              }
            }
          }
        }
        n171 = Bundle By Name(cluster=T3 {"L1 PID Gains"={"Kp"=0.005, "Kd"=0.5, "Ki"=0.0005}, "L2 PID Gains"={"Kp"=0.01, "Kd"=1.0, "Ki"=0.0005}, "L3 PID Gains"={"Kp"=0.05, "Kd"=1.0, "Ki"=0.0005}, "L4 PID Gains"={"Kp"=0.1, "Kd"=1.0, "Ki"=0.0005}} ("L1 to L4 PID Cluster 2"), "L1 PID Gains"="L1 PID Gains", "L2 PID Gains"="L2 PID Gains", "L3 PID Gains"="L3 PID Gains", "L4 PID Gains"="L4 PID Gains") -> (→"L1 to L4 PID Cluster":T3)
        n172 = Bundle By Name(cluster=T2 {"Stage Z PID"={"Kp"=0.0005, "Kd"=0.001, "Ki"=0.0}, "Stage Y PID"={"Kp"=0.0003, "Kd"=0.01, "Ki"=0.0}, "Stage X PID"={"Kp"=0.0003, "Kd"=0.01, "Ki"=0.0}} ("Stage PID Cluster 2"), "Stage X PID"="Stage X PID Gains", "Stage Y PID"="Stage Y PID Gains", "Stage Z PID"="Stage Z PID Gains") -> (→"Stage PID Cluster":T2)
        n173 = global write "Global Variables.vi" "L4 M/S cmd"("L4 [deg]") -> ()
        n174 = local read "Program Stop"() -> (w292:bool)
        n175 = Or(x="L3 Go Home", y=w292) -> (x .or. y?=w293:bool)
        n176 = global write "Global Variables.vi" "pause"("Pause") -> ()
        n177 = global write "Global Variables.vi" "reset joystick"("Reset Joystick") -> ()
        n178 = global write "Global Variables.vi" "L3 go home"(w293) -> ()
        n179 = global write "Global Variables.vi" "stop accurus"("Stop Accurus") -> ()
        n180 = global write "Global Variables.vi" "irrigate"("Irrigation") -> ()
        n181 = case shown="False" "PID ON/OFF" {
          frame False {
            n182 = property on="Vac Cmd" class="DigNum (strict)"("DisabledEnum"=T13."Enabled" ("Disabled")) -> ()  [unwired: 2 in, 2 out]
          }
          frame True {
            n183 = property on="Vac Cmd" class="DigNum (strict)"("DisabledEnum"=T13."Disabled" ("Disabled")) -> ()  [unwired: 2 in, 2 out]
          }
        }
        n184 = global write "Global Variables.vi" "joint limits"("Joint Limits") -> ()
        n185 = global write "Global Variables.vi" "octDir"("OCT Direction") -> ()
        n186 = flat-sequence {
          frame #0 {
            n187 = call "RisingEdge.vi"("Signal In"="Take IOP Data") -> ("Rising Edge"=w309:bool)  [unwired: 10 in]
            n188 = case shown="True" w309 {
              selector: w309 -> [_ w311]
              frame False {
              }
              frame True {
                n189 = global write "Global Variables.vi" "take IOP data"(w311) -> ()
              }
            }
          }
          frame #1 {
            n190 = local write "Take IOP Data"(FALSE ("Take IOP Data")) -> ()
          }
        }
        n191 = global write "Global Variables.vi" "program stop"("Program Stop") -> ()
      }
      n192 = while {
        stop <- w146 stop-if-true
        # "Indicator Loop"
        n193 = Wait (ms)(milliseconds to wait=u32 100) -> ()  [unwired: 1 out]
        n194 = global read "Global Variables.vi" "L1 to L4 cmd Posit"() -> (w138:dbl[])
        n195 = global read "Global Variables.vi" "L1 to L4 out Posit"() -> (w141:dbl[])
        n196 = Index Array(array=w141, index #1=0 ("index"), index #2=1 ("index"), index #3=2 ("index"), index #4=3 ("index")) -> (element #1=w144:dbl, element #2=w143:dbl, element #3=w142:dbl, element #4=→"L4 out Posit":dbl)
        "L3 out Posit" <- w142
        "L2 out Posit" <- w143
        "L1 out Posit" <- w144
        n197 = Index Array(array=w138, index #1=0 ("index"), index #2=1 ("index"), index #3=2 ("index"), index #4=3 ("index")) -> (element #1=w120:dbl, element #2=w119:dbl, element #3=w118:dbl, element #4=→"L4 cmd Posit" →"L4 Chart":dbl)
        "L1 cmd Posit" <- w120
        "L3 cmd Posit" <- w118
        "L2 cmd Posit" <- w119
        "L2 Chart" <- w119
        "L1 Chart" <- w120
        "L3 Chart" <- w118
        n198 = call "Forward_Kinematics_v2.vi"("theta 3"=w118, "theta 2"=w119, "theta 1"=w120) -> ("position"=→"Tip cmd Posit":dbl[])
        n199 = call "Forward_Kinematics_v2.vi"("theta 3"=w142, "theta 2"=w143, "theta 1"=w144) -> ("position"=w133:dbl[])
        "Tip out Posit" <- w133
        n200 = shared-variable "PXI-Robot\\JointAngles.lvlib\\ToolTipPosition"(w133) -> ()  [unwired: 1 in, 1 out]
        n201 = disable-structure shown="Disabled" {
          frame Disabled {
            n202 = global read "Global Variables.vi" "Accurus cluster"() -> (w172:T15)
            n203 = Unbundle By Name(w172) -> ("Accurus engaged?"=→"Accurus Engaged?":bool, "Accurus button"=→"Accurus Button":bool[], "Accurus Ch. A Vout"=→"Voltage Output Ch. A":dbl, "Accurus Ch. B Vout"=→"Voltage Output Ch. B":dbl, "Vacuum Force"=→"Vacuum Force [mmHg]" →"Vacuum Force [mmHg]  2":i32, "Irrigation engaged?"=→"Irrigation Engaged?" →"Irrigation Engaged? 2":bool)
          }
          frame Enabled {
          }
        }
        n204 = global read "Global Variables.vi" "Stage cmd Posit"() -> (w139:dbl[])
        n205 = global read "Global Variables.vi" "Stage out Posit"() -> (w140:dbl[])
        n206 = Index Array(array=w140, index #1=0 ("index"), index #2=1 ("index"), index #3=2 ("index")) -> (element #1=→"X Stage out [mm]" →"X Stage out [mm] 2":dbl, element #2=→"Y Stage out [mm]" →"Y Stage out [mm] 2":dbl, element #3=→"Z Stage out [mm]" →"Z Stage out [mm] 2":dbl)
        n207 = Index Array(array=w139, index #1=0 ("index"), index #2=1 ("index"), index #3=2 ("index")) -> (element #1=→"X Stage cmd [mm]":dbl, element #2=→"Y Stage cmd [mm]":dbl, element #3=→"Z Stage cmd [mm]":dbl)  [unwired: 1 in, 1 out]
        n208 = global read "Global Variables.vi" "state flag array"() -> (→"State Flag Array":bool[])
        n209 = global read "Global Variables.vi" "state changing"() -> (→"State changing":bool)
        n210 = global read "Global Variables.vi" "OCT Z cmd Posit"() -> (→"OCT Z cmd [mm]":dbl)
        n211 = global read "Global Variables.vi" "OCT Z out Posit"() -> (→"OCT Z out [mm]":dbl)
        n212 = local read "Target IOP"() -> (w124:sgl)
        n213 = local read "Vac Cmd"() -> (w125:sgl)
        n214 = local read "Pressure Reading"() -> (w116:dbl[])
        n215 = global read "Global Variables.vi" "current run no."() -> (→"Current No.":u8)
        n216 = global read "Global Variables.vi" "finished late counts"() -> (→"Finished Late Counts":u16)
        n217 = Index Array(array=w116, index #1=0 ("index"), index #2=1 ("index"), index #3=2 ("index"), index #4=3 ("index")) -> (element #1=→"Vacuum":dbl, element #2=→"Irrigation":dbl, element #3=w110:dbl)  [unwired: 1 out]
        "AC Pressure [mmHg]" <- w110
        n218 = Build Array(w124, w110, w125) -> (w123:dbl[])
        n219 = Array To Cluster(array=w123) -> (cluster=→"IOP Ctrl":T6)
        n220 = Array To Cluster(array=w116) -> (cluster=→"Pressure Sensors":T7)
        n221 = case shown="True" "Clear Charts" {
          frame False {
          }
          frame True {
            w173 = T16 [] ("History Data")
            n222 = property on="IOP Ctrl" class="WFChart (strict)"("History Data"=w173) -> ()  [unwired: 2 in, 2 out]
            n223 = property on="Pressure Sensors" class="WFChart (strict)"("History Data"=w173) -> ()  [unwired: 2 in, 2 out]
          }
        }
        n224 = local read "Program Stop"() -> (w146:bool)
      }
      n225 = node-c288(w34) -> ()  [unwired: 1 out]
      n226 = Build Array(w37, w37, w37, w37, w37, w37, w37, w37) -> (w43:i16[])
      n227 = xnode "Output Shut Down"("FPGA VI Reference In"=w42, "error in"=w41, "AO"=w43, "INHB X"=w44, "INHB Y"=w44, "INHB Z"=w44, "INHB OCT Mot"=w44) -> ("FPGA VI Reference Out"=w39:refnum<k20>, "error out"=w40:errorcluster)
    }
    frame #2 {
      n228 = xnode "FPGA Reset"("FPGA VI Reference In"=w396, "error in"=w395) -> ("FPGA VI Reference Out"=w399:refnum<k20>, "error out"=w398:errorcluster)
      n229 = xnode "Close FPGA VI Reference"("FPGA VI Reference In"=w399, "error in"=w398) -> ("error out"=→"Error(s) Out on Program End":errorcluster)
    }
  }
